vi "Write Message (Serial).vi"(6 "options":T1={"ignore timeout error"=TRUE, "timeout ms (1000)"=1000}, 8 "error in":errorcluster, 9 "data":string, 10 "name":string, 11 "connection info in":T2) -> (0 "error out":errorcluster, 3 "connection info out":T2)   [LabVIEW 2010, in "NI STM.lvlib"]
doc: "This VI writes a package of data to a remote computer. It prepends a meta data ID number to each packet. \n\nThe data must be passed in as a String. The calling VI is responsible for flattening the desired data to a string before passing it to this VI. \n\n\nCopyright 2015, 2016, 2017 National Instruments Corporation\n\nLicensed under the Apache License, Version 2.0 (the \"License\"); you may not use this file except in compliance with the License.\n\n You may obtain a copy of the License at\n\n http://www.apache.org/licenses/LICENSE-2.0\n\nUnless required by applicable law or agreed to in writing, software distributed under the License is distributed on an \"AS IS\" BASIS, WITHOUT WARRANTIES OR CONDITIONS OF ANY KIND, either express or implied.\n\nSee the License for the specific language governing permissions and limitations under the License."
uses:
  NI STM.lvlib
  Serial Connection Info.ctl
  SubVIs/MetaDataElement.ctl
  Serial Write Options.ctl
  SubVIs/GetIDfromName.vi
  SubVIs/Generate STM Error.vi
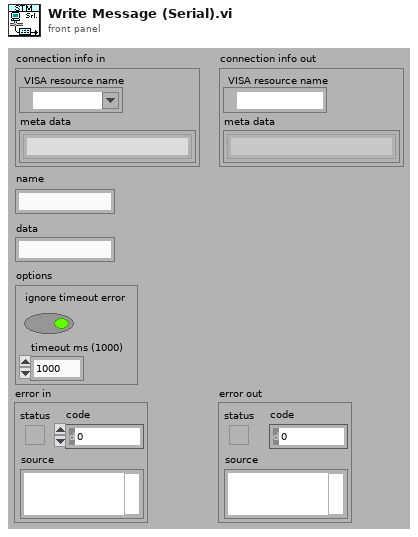
[diagram p1: front panel]
types:
  T1 = typedef "NI STM.lvlib/Serial Write Options.ctl" = cluster{"ignore timeout error":bool, "timeout ms (1000)":u32}
  T2 = typedef "NI STM.lvlib/Serial Connection Info.ctl" = cluster{"VISA resource name":refnum<visa-resource-name>, "meta data":T3[]}
  T3 = typedef "NI STM.lvlib/MetaDataElement.ctl" = string
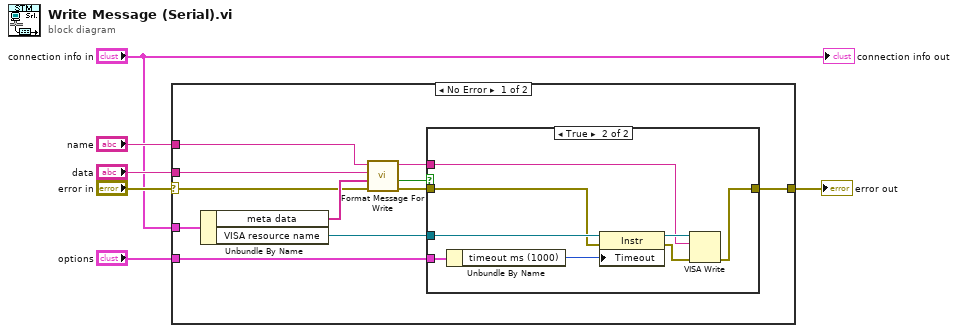
[diagram p0: block diagram]
diagram:
  n1 = case shown="No Error" "error in" {
    selector: "error in" -> [w11 w27]
    tunnel: "connection info in" -> [w15 _]
    tunnel: [w17 w27] -> w6
    tunnel: "name" -> [w14 _]
    tunnel: "data" -> [w13 _]
    tunnel: "options" -> [w7 _]
    frame No Error {
      n2 = Unbundle By Name(w15) -> ("meta data"=w12:T3[], "VISA resource name"=w16:refnum<visa-resource-name>)
      n3 = call "Format Message For Write.vi"("error in"=w11, "meta data"=w12, "data"=w13, "message name"=w14) -> ("error out"=w10:errorcluster, "valid?"=w9:bool, "message"=w8:string)  [unwired: 5 in]
      n4 = case shown="True" w9 {
        tunnel: w16 -> [_ w25]
        tunnel: w10 -> [w18 w21]
        tunnel: [w18 w26] -> w17
        tunnel: w8 -> [_ w22]
        tunnel: w7 -> [_ w19]
        frame False {
        }
        frame True {
          n5 = Unbundle By Name(w19) -> ("timeout ms (1000)"=w20:u32)
          n6 = property class="Instr"(reference=w25, error in=w21, "Timeout"=w20) -> (reference out=w23:refnum<visa-resource-name>, error out=w24:errorcluster)
          n7 = VISA Write(VISA resource name=w23, write buffer=w22, error in (no error)=w24) -> (error out=w26:errorcluster)  [unwired: 2 out]
        }
      }
    }
    frame Error {
    }
  }
  "error out" <- w6
  "connection info out" <- "connection info in"
